vi "key_char_check.vi"(8 "key value[1]":dbl, 9 "keys pressed[1]":dbl, 10 "key value[0]":dbl, 11 "keys pressed[0]":dbl) -> (2 "control":bool)   [LabVIEW 2011]
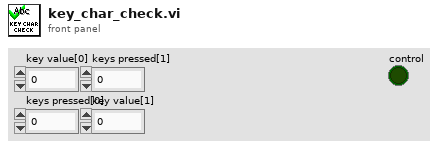
[diagram p1: front panel]
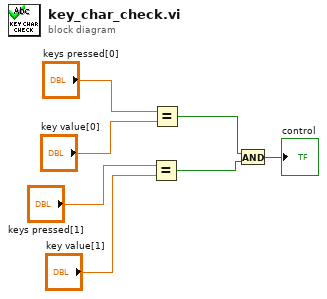
[diagram p0: block diagram]
diagram:
  n1 = Equal?(x="keys pressed[1]", y="key value[1]") -> (x = y?=w6:bool)
  n2 = Equal?(x="keys pressed[0]", y="key value[0]") -> (x = y?=w7:bool)
  n3 = And(x=w7, y=w6) -> (x .and. y?=→"control":bool)
